vi "Calibrate Current Sense Resistiviy_BU.vi"(0 "DMM ref in":refnum<visa-resource-name>="USB0::0x2A8D::0x0101::MY59004074::INSTR", 3 "Calibrate Stop 2":refnum<vi>, 5 "DMM error in":errorcluster, 7 "Channel  Count":i32, 8 "Current Sense \nResitance Array\nREF":refnum<vi>, 9 "ESP32 ref in":refnum<visa-resource-name>="COM4", 11 "ESP32 error in":errorcluster, 14 "Time out count REF":refnum<vi>) -> (10 "ESP32 ref out":refnum<visa-resource-name>, 15 "ESP32 error out":errorcluster)   [LabVIEW 2023]
uses:
  <instrlib>/Agilent 3446X Series/Agilent 3446X Series.lvlib
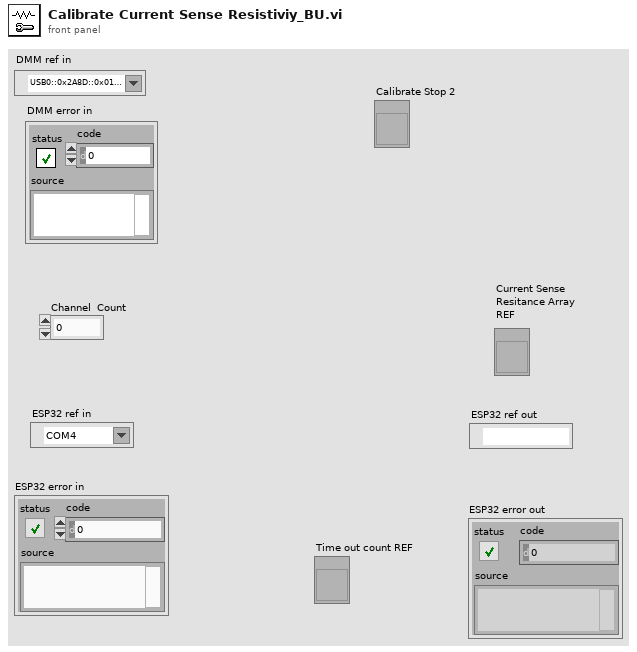
[diagram p1: front panel]
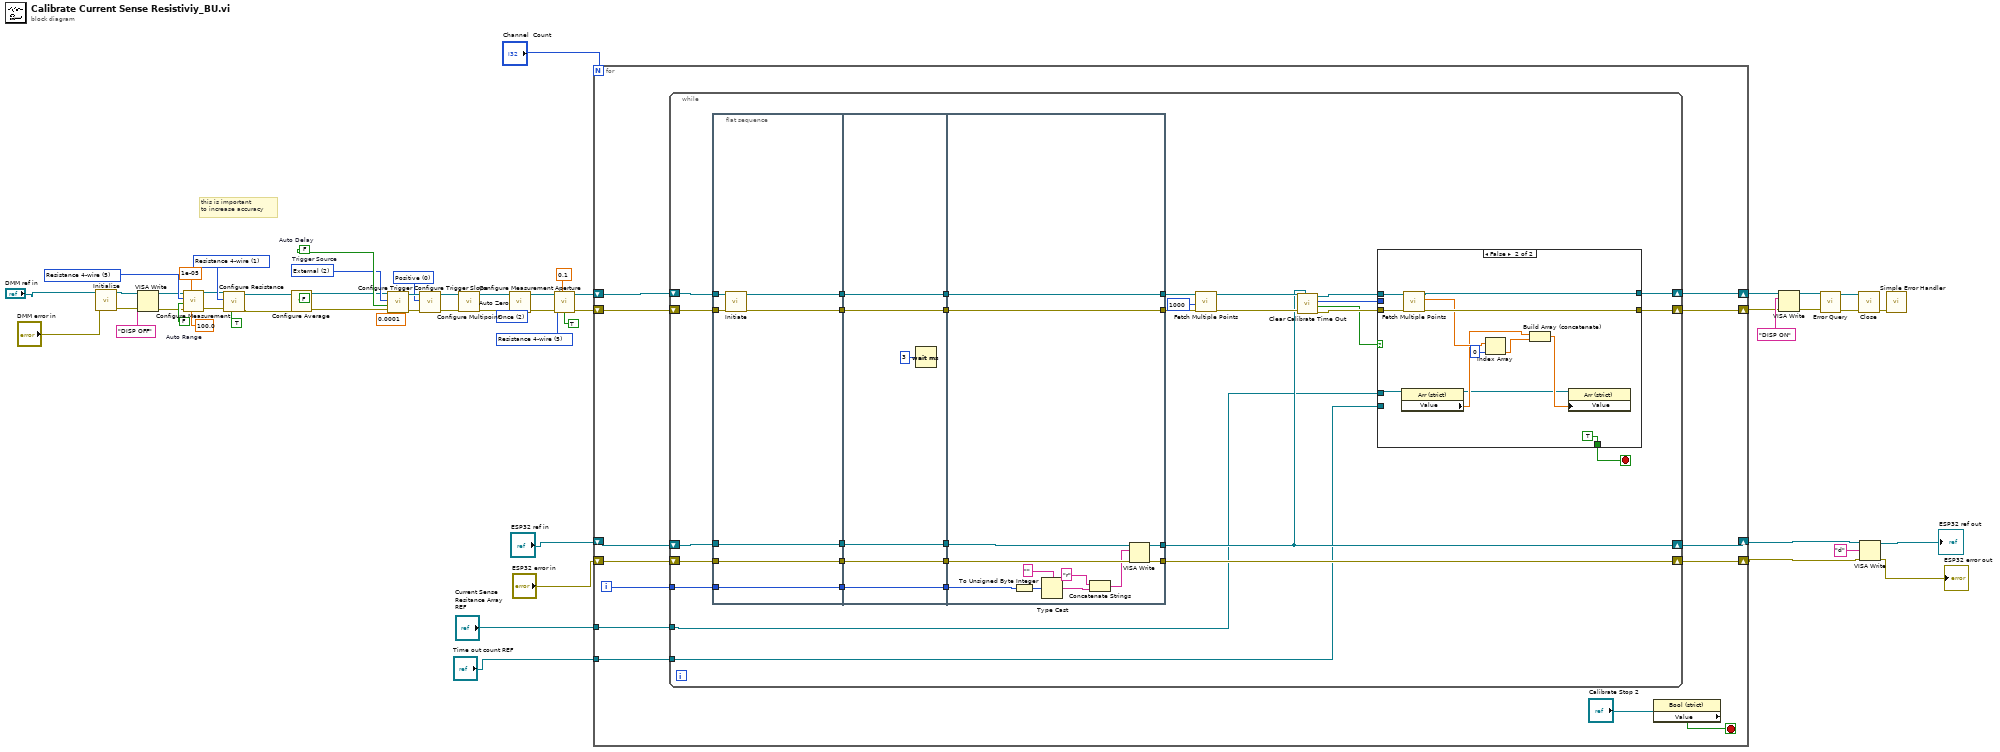
[diagram p0: block diagram]
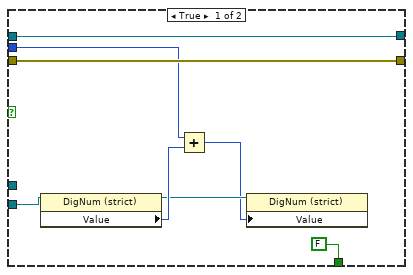
[diagram p2: hidden frame]
diagram:
  w35 = 0 items=["Positive", "Negative"] ("Trigger Edge (1: Negative)")
  w32 = 2 items=["Immediate", "Software (Bus)", "External"]  # Trigger Source
  w34 = FALSE  # Auto Delay
  w43 = 5 items=["Continuity", "Current AC", "Current DC", "Diode", "Frequency", "Resistance 4-wire", "Period", "Resistance 2-wire", "Temperature", "Voltage AC", "Voltage DC", "Voltage DC Ratio", "Capacitance"] ("Measurement Function (10: Voltage DC)")
  w47 = 1 items=["Resistance 2-wire", "Resistance 4-wire"] ("Resistance Type (0: Resistance 2-wire)")
  w49 = 5 items=["Continuity", "Current AC", "Current DC", "Diode", "Frequency", "Resistance 4-wire", "Period", "Resistance 2-wire", "Temperature", "Voltage AC", "Voltage DC", "Voltage DC Ratio", "Capacitance"] ("Measurement Function (0: Continuity)")
  w53 = 2 items=["Disable", "Enable", "Once"] ("Auto Zero (1: Enable)")
  w56 = FALSE  # Auto Range
  # "this is important \nto increase accuracy"
  n1 = call <instrlib>:"Initialize.vi"("error in (no error)"="DMM error in", "VISA resource name"="DMM ref in") -> ("error out"=w18:errorcluster, "VISA resource name out"=w20:refnum<visa-resource-name>)  [unwired: 3 in, 5 out]
  n2 = VISA Write(VISA resource name=w20, write buffer="DISP OFF", error in (no error)=w18) -> (VISA resource name out=w19:refnum<visa-resource-name>, error out=w17:errorcluster)  [unwired: 1 out]
  n3 = call <instrlib>:"Configure Measurement.vi"("Manual Range (1)"=100.0, "Absolute Resolution (1E-6)"=1e-05, "error in (no error)"=w17, "Auto Range (T: Enable)"=w56, "Measurement Function (10: Voltage DC)"=w43, "VISA resource name"=w19) -> ("error out"=w44:errorcluster, "VISA resource name out"=w45:refnum<visa-resource-name>)  [unwired: 4 out]
  n4 = call <instrlib>:"Configure Resistance.vi"("Enable Offset Compensation (F: Disable)"=TRUE, "error in (no error)"=w44, "Resistance Type (0: Resistance 2-wire)"=w47, "VISA resource name"=w45) -> ("error out"=w29:errorcluster, "VISA resource name out"=w30:refnum<visa-resource-name>)  [unwired: 6 in]
  n5 = call <instrlib>:"Configure Average.vi"("error in (no error)"=w29, "Enable Statistics (F: Disable)"=FALSE, "VISA resource name"=w30) -> ("error out"=w27:errorcluster, "VISA resource name out"=w28:refnum<visa-resource-name>)  [unwired: 7 in]
  n6 = call <instrlib>:"Configure Trigger.vi"("Manual Trigger Delay (1 s)"=0.0001, "error in (no error)"=w27, "Auto Delay (F:Disable)"=w34, "Trigger Source (0: Immediate)"=w32, "VISA resource name"=w28) -> ("error out"=w37:errorcluster, "VISA resource name out"=w36:refnum<visa-resource-name>)  [unwired: 1 in, 4 out]
  n7 = call <instrlib>:"Configure Trigger Slope.vi"("error in (no error)"=w37, "Trigger Edge (1: Negative)"=w35, "VISA resource name"=w36) -> ("error out"=w25:errorcluster, "VISA resource name out"=w26:refnum<visa-resource-name>)  [unwired: 7 in]
  n8 = call <instrlib>:"Configure Multipoint.vi"("error in (no error)"=w25, "VISA resource name"=w26) -> ("error out"=w23:errorcluster, "VISA resource name out"=w24:refnum<visa-resource-name>)  [unwired: 5 in, 3 out]
  n9 = call <instrlib>:"Auto Zero.vi"("error in (no error)"=w23, "Auto Zero (1: Enable)"=w53, "VISA resource name"=w24) -> ("error out"=w52:errorcluster, "VISA resource name out"=w51:refnum<visa-resource-name>)  [unwired: 7 in]
  n10 = call <instrlib>:"Configure Measurement Aperture.vi"("Aperture Time (0.1s)"=0.1, "error in (no error)"=w52, "Enable Aperture (F: Disable)"=TRUE, "Measurement Function (0: Continuity)"=w49, "VISA resource name"=w51) -> ("error out"=w41:errorcluster, "VISA resource name out"=w42:refnum<visa-resource-name>)  [unwired: 5 in]
  n11 = for {
    N: "Channel  Count" -> [_]
    shift-right: [w67] -> w4
    shift-left: "ESP32 ref in" -> [w69]
    shift-right: [w66] -> w3
    shift-left: "ESP32 error in" -> [w68]
    shift-right: [w61] -> w5
    shift-left: w41 -> [w63]
    shift-right: [w62] -> w6
    shift-left: w42 -> [w64]
    tunnel: "Current Sense \nResitance Array\nREF" -> [w60]
    tunnel: "Time out count REF" -> [w59]
    i -> [w65]
    stop <- w57 stop-if-true
    n12 = while {
      tunnel: w65 -> [w87]
      shift-right: [w73] -> w67
      shift-left: w69 -> [w90]
      shift-right: [w88] -> w66
      shift-left: w68 -> [w89]
      shift-right: [w84] -> w62
      shift-left: w64 -> [w86]
      shift-right: [w83] -> w61
      shift-left: w63 -> [w85]
      tunnel: w60 -> [w72]
      tunnel: w59 -> [w70]
      stop <- w79 stop-if-true
      n13 = flat-sequence {
        tunnel: w87 -> [w125]
        tunnel: w89 -> [w126]
        tunnel: w90 -> [w127]
        tunnel: [w127] -> w100
        tunnel: [w126] -> w99
        tunnel: [w125] -> w98
        tunnel: w86 -> [w124]
        tunnel: w85 -> [w123]
        tunnel: [w122] -> w97
        tunnel: [w121] -> w96
        tunnel: [w133] -> w95
        tunnel: [w132] -> w94
        tunnel: [w131] -> w93
        tunnel: w100 -> [w133]
        tunnel: w99 -> [w132]
        tunnel: w98 -> [w131]
        tunnel: [w130] -> w92
        tunnel: w97 -> [w130]
        tunnel: [w129] -> w91
        tunnel: w96 -> [w129]
        tunnel: [w143] -> w73
        tunnel: [w139] -> w88
        tunnel: w95 -> [w145]
        tunnel: w94 -> [w144]
        tunnel: w93 -> [w137]
        tunnel: [w136] -> w78
        tunnel: w92 -> [w136]
        tunnel: [w135] -> w77
        tunnel: w91 -> [w135]
        frame #0 {
          n14 = call <instrlib>:"Initiate.vi"("error in (no error)"=w123, "VISA resource name"=w124) -> ("error out"=w121:errorcluster, "VISA resource name out"=w122:refnum<visa-resource-name>)  [unwired: 8 out]
        }
        frame #1 {
          n15 = Wait (ms)(milliseconds to wait=u32 3) -> ()  [unwired: 1 out]
        }
        frame #2 {
          n16 = To Unsigned Byte Integer(number=w137) -> (unsigned 8bit integer=w140:u8)
          n17 = Type Cast(type="" ("string"), x=w140) -> (*(type *) &x=w138:string)
          n18 = Concatenate Strings("r" ("data in"), w138) -> (w134:string)
          n19 = VISA Write(VISA resource name=w145, write buffer=w134, error in (no error)=w144) -> (VISA resource name out=w143:refnum<visa-resource-name>, error out=w139:errorcluster)  [unwired: 1 out]
        }
      }
      n20 = call <instrlib>:"Fetch Multiple Points.vi"("error in (no error)"=w77, "Timeout (10000 ms)"=1000, "VISA resource name"=w78) -> ("error out"=w75:errorcluster, "VISA resource name out"=w76:refnum<visa-resource-name>)  [unwired: 1 in, 6 out]
      n21 = call "Clear Calibrate Time Out.vi"("VISA resource name"=w73, "error in (no error)"=w75, "VISA Refnum in"=w76) -> ("error out"=w81:errorcluster, "error?"=w80:bool, "Time out count"=w71:i32, "VISA Refnum out"=w82:refnum<visa-resource-name>)  [unwired: 5 in]
      n22 = case shown="False" w80 {
        tunnel: [w107 w120] -> w84
        tunnel: [w106 w119] -> w83
        tunnel: w82 -> [w107 w115]
        tunnel: w81 -> [w106 w114]
        tunnel: [FALSE TRUE] -> w79
        tunnel: w72 -> [_ w111]
        tunnel: w71 -> [w105 _]
        tunnel: w70 -> [w104 _]
        frame True {
          n23 = property class="DigNum (strict)"(reference=w104) -> (reference out=w102:refnum<vi>, "Value"=w103:i32)  [unwired: 1 in, 1 out]
          n24 = Add(x=w105, y=w103) -> (x+y=w101:i32)
          n25 = property class="DigNum (strict)"(reference=w102, "Value"=w101) -> ()  [unwired: 1 in, 2 out]
        }
        frame False {
          n26 = property class="Arr (strict)"(reference=w111) -> (reference out=w109:refnum<vi>, "Value"=w112:dbl[])  [unwired: 1 in, 1 out]
          n27 = call <instrlib>:"Fetch Multiple Points.vi"("error in (no error)"=w114, "VISA resource name"=w115) -> ("error out"=w119:errorcluster, "Measurements"=w118:dbl[], "VISA resource name out"=w120:refnum<visa-resource-name>)  [unwired: 7 in]
          n28 = Index Array(array=w118, index=0) -> (element=w117:dbl)
          n29 = Build Array (concatenate)(w112, w117) -> (w110:dbl[])
          n30 = property class="Arr (strict)"(reference=w109, "Value"=w110) -> ()  [unwired: 1 in, 2 out]
        }
      }
    }
    n31 = property class="Bool (strict)"(reference="Calibrate Stop 2") -> ("Value"=w57:bool)  [unwired: 1 in, 2 out]
  }
  n32 = VISA Write(VISA resource name=w6, write buffer="DISP ON", error in (no error)=w5) -> (VISA resource name out=w15:refnum<visa-resource-name>, error out=w14:errorcluster)  [unwired: 1 out]
  n33 = call <instrlib>:"Error Query.vi"("error in (no error)"=w14, "VISA resource name"=w15) -> ("error out"=w40:errorcluster, "VISA resource name out"=w39:refnum<visa-resource-name>)  [unwired: 8 out]
  n34 = call <instrlib>:"Close.vi"("error in (no error)"=w40, "VISA resource name"=w39) -> ("error out"=w38:errorcluster)  [unwired: 9 out]
  n35 = VISA Write(VISA resource name=w4, write buffer="d" ("data in"), error in (no error)=w3) -> (VISA resource name out=→"ESP32 ref out":refnum<visa-resource-name>, error out=→"ESP32 error out":errorcluster)  [unwired: 1 out]
  n36 = call <vilib>:"Simple Error Handler.vi"("error in (no error)"=w38) -> ()  [unwired: 1 in, 8 out]
